vi "VITester_Global_Interface.vi"() -> (3 "InterfaceTable":T1)   [LabVIEW 2013]
uses:
  <resource>/Framework/Providers/API/Global_Interface.ctl
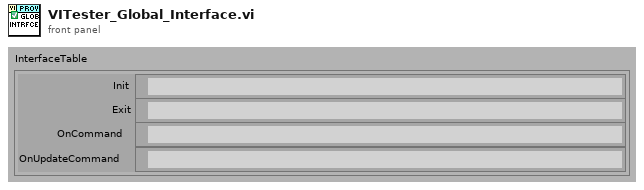
[diagram p1: front panel]
types:
  T1 = typedef "Global_Interface.ctl" = cluster{"Init":path, "Exit":path, "OnCommand":path, "OnUpdateCommand":path}
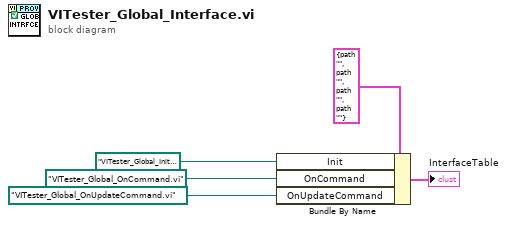
[diagram p0: block diagram]
diagram:
  n1 = Bundle By Name(cluster=T1 {"Init"=path "", "Exit"=path "", "OnCommand"=path "", "OnUpdateCommand"=path ""} ("InterfaceTable"), "Init"=path "VITester_Global_Init.vi", "OnCommand"=path "VITester_Global_OnCommand.vi", "OnUpdateCommand"=path "VITester_Global_OnUpdateCommand.vi") -> (→"InterfaceTable":T1)
